vi "Get Notifiers.vi"(8 "error in (no error)":errorcluster, 10 "Notifier of Notifiers":refnum<notifier>, 11 "PID Loop in":refnum<class "PID Loop.lvclass">) -> (0 "error out":errorcluster, 3 "PID Loop out":refnum<class "PID Loop.lvclass">)   [LabVIEW 2024, in "PID Loop.lvlib" / "PID Loop.lvclass"]
uses:
  PID Loop.lvclass
  PID Loop.lvclass/PID Loop.ctl
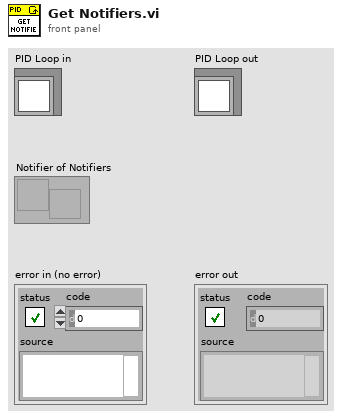
[diagram p1: front panel]
types:
  T1 = cluster{"Setpoint Notifier":refnum<notifier>, "Process Variable Notifier":refnum<notifier>, "Output Notifier":refnum<notifier>}
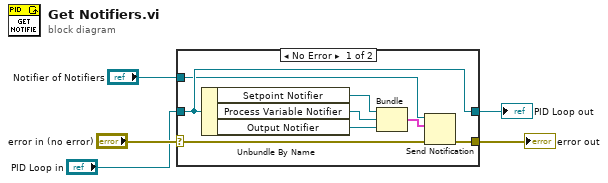
[diagram p0: block diagram]
diagram:
  n1 = case shown="No Error" "error in (no error)" {
    selector: "error in (no error)" -> [w7 w15]
    tunnel: [w6 w15] -> w4
    tunnel: [w13 w14] -> w2
    tunnel: "PID Loop in" -> [w13 w14]
    tunnel: "Notifier of Notifiers" -> [w9 _]
    frame No Error {
      n2 = Unbundle By Name(w13) -> ("Setpoint Notifier"=w12:refnum<notifier>, "Process Variable Notifier"=w11:refnum<notifier>, "Output Notifier"=w10:refnum<notifier>)
      n3 = Bundle("Setpoint Notifier"=w12, "Process Variable Notifier"=w11, "Output Notifier"=w10) -> (w8:T1)  [unwired: 1 in]
      n4 = Send Notification(notification=w8, notifier=w9, error in (no error)=w7) -> (error out=w6:errorcluster)  [unwired: 1 out]
    }
    frame Error {
    }
  }
  "error out" <- w4
  "PID Loop out" <- w2
